vi "Actor Core.vi"(8 "error in":errorcluster, 11 "Nested in":refnum<class "Object Dictionary.lvclass">) -> (0 "error out":errorcluster, 3 "Actor out":refnum<class "Actor.lvclass">)   [LabVIEW 2024, in "Object Dictionary.lvlib" / "Object Dictionary.lvclass"]
doc: "(<B>Filename</B>: Actor Framework.lvlib:Actor.lvclass:Actor Core.vi)\n\nReceives messages to the actor, reacts to them, and initiates any error handling that may shut the actor down.\n\nDescendant classes may override this VI to append parallel tasks for the actor to complete while it handles messages. Overrides use the Call Parent Method node."
uses:
  Object Dictionary.lvclass
  <vilib>/ActorFramework/Actor/Actor.lvclass
  Object Dictionary.lvclass/Object Dictionary.ctl
  <vilib>/ActorFramework/Message Enqueuer/Message Enqueuer.lvclass/Message Enqueuer.ctl
  <vilib>/ActorFramework/Message Enqueuer/Enqueue.vi
  <vilib>/ActorFramework/Stop Msg/Stop Msg.lvclass
  <vilib>/Utility/LVClass/Get LV Class Name.vi
  <resource>/AFDebug/Generate Trace for Message.vi
  <vilib>/ActorFramework/Message Priority Queue/Priority Enqueue.vi
  <vilib>/MGI/Panel Manager/Panel Actor/Panel Actor/Panel Actor.lvclass
types:
  T1 = cluster{"Pnl Actor":refnum<event-registration>, "Event Registration Refnum":refnum<event-registration>}
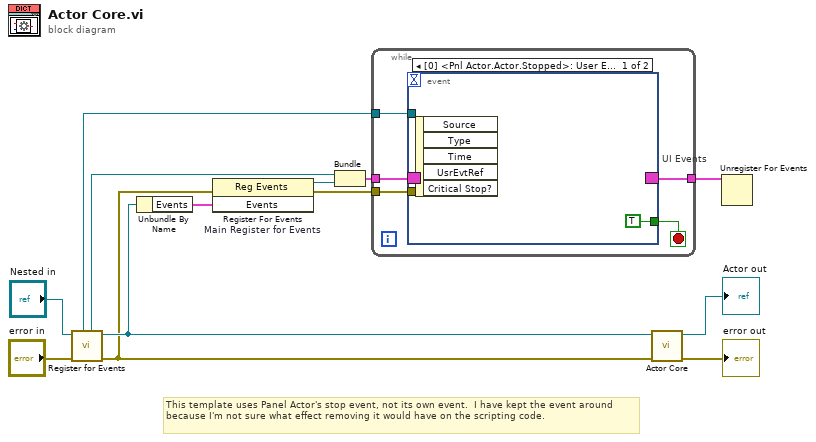
[diagram p0: block diagram]
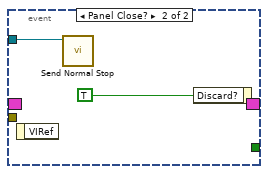
[diagram p2: hidden frame]
diagram:
  # "This template uses Panel Actor's stop event, not its own event.  I have kept the event around because I'm not sure what effect removing it would have on the scripting code."
  n1 = call <vilib>:"Register for Events.vi"("Error In"="error in", "Panel Actor in"="Nested in") -> ("Error Out"=w2:errorcluster, "Panel Actor out"=w6:refnum<class "Object Dictionary.lvclass">, "Pnl Actor"=w3:refnum<event-registration>, "Self Enqueuer"=w5:refnum<class "Message Enqueuer.lvclass">)  [unwired: 6 in]
  n2 = Unbundle By Name(w6) -> ("Events"=w10:cluster{"None":refnum<user-event>})
  n3 = register-events "Main Register for Events"(error in=w2, w10) -> (reference out=w11:refnum<event-registration>, error out=w1:errorcluster)  [unwired: 1 in]
  n4 = Bundle("Pnl Actor"=w3, "Event Registration Refnum"=w11) -> (w4:T1)  [unwired: 1 in]
  n5 = while {
    tunnel: w4 -> [w18]
    tunnel: [w16] -> w9
    tunnel: w5 -> [w15]
    tunnel: w1 -> [w14]
    stop <- w17 stop-if-true
    n6 = event "UI Events" shown="[0] <Pnl Actor.Actor.Stopped>: User Event" {
      selector: w18 -> [_ _]
      dyn-events: [_ _] -> w16
      timeout: _ -> [_ _]
      tunnel: [TRUE _] -> w17
      tunnel: w15 -> [_ w20]
      tunnel: w14 -> [_ _]
      event User Event {
        n7 = event-data() -> ()  [unwired: 1 in, 5 out]
      }
      event Panel Close? {
        n8 = event-data() -> ()  [unwired: 1 in, 1 out]
        n9 = call <vilib>:"Send Normal Stop.vi"("Message Enqueuer"=w20) -> ()  [unwired: 10 in, 1 out]
        n10 = event-data("Discard?"=TRUE) -> ()  [unwired: 1 in, 1 out]
      }
    }
  }
  n11 = call-parent "Actor Core.vi"("error in"=w2, "Panel Actor in"=w6) -> ("error out"=→"error out":errorcluster, "Actor out"=→"Actor out":refnum<class "Actor.lvclass">)  [unwired: 8 in]
  n12 = Unregister For Events(event registration refnum=w9) -> ()  [unwired: 1 in, 1 out]
